vi "Stop AsyncThread LowLevel.vi"(8 "error in":errorcluster, 10 "Handle":u64, 11 "path in":path) -> (0 "error out":errorcluster, 3 "dup path":path)   [LabVIEW 2016, in "DemoSkeleton.lvlib"]
uses:
  DemoSkeleton.lvlib
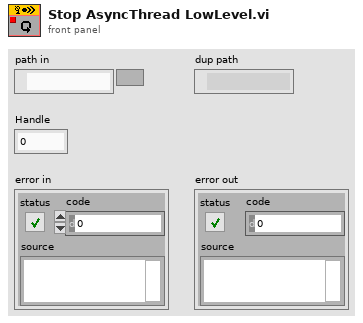
[diagram p1: front panel]
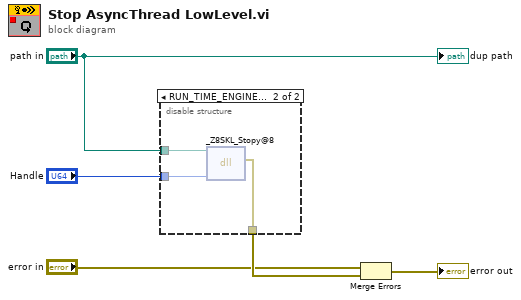
[diagram p0: block diagram]
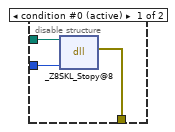
[diagram p2: hidden frame]
diagram:
  n1 = disable-structure shown="RUN_TIME_ENGINE==True" {
    disable-tunnel: [w8 w11] -> w4
    disable-tunnel: "Handle" -> [w7 w10]
    disable-tunnel: "path in" -> [w6 w9]
    frame condition #0 (active) {
      n2 = dll-call lib="C:/Users/loic.wohleber/Desktop/PostLVUserEvent_Demo/Sources/LabVIEW/Library/DemoSkeleton/skeleton_lv_event_lv.dll" fn="_Z8SKL_Stopy@8" label="Stop"(path in=w6, "Handle"=w7) -> (error out=w8:errorcluster)  [unwired: 4 in, 1 out]
    }
    frame condition #1 {
      n3 = dll-call lib="C:/Users/loic.wohleber/Desktop/PostLVUserEvent_Demo/Sources/LabVIEW/Library/DemoSkeleton/skeleton_lv_event_lvrt.dll" fn="_Z8SKL_Stopy@8" label="StopRT"(path in=w9, "Handle"=w10) -> (error out=w11:errorcluster)  [unwired: 4 in, 1 out]
    }
  }
  n4 = Merge Errors("error in", w4) -> (→"error out":errorcluster)
  "dup path" <- "path in"
